vi "GetActivePortNames.vi"(0 "Channel Properties":T1[](array[typedef]) {"Current Pos" format="%.2f"; "Backlash/Eng units" format="%.2f"; "Pulses/rev" format="%.2f"; "Pos Tolerance" format="%.2f"; "Pulses/unit" format="%.2f"; "Acc. Min" format="%.2f"; "Acc. Max" format="%.2f"; "Vel. Min" format="%.2f"; "Vel. Max" format="%.2f"; "Acc. Default" format="%.2f"; "Vel. Default" format="%.2f"}) -> (1 "Port Name Array":string[](array[string]), 2 "Drive Type Array":T2[](array[typedef]), 3 "Address":u8[](array[numeric]))   [LabVIEW 2022 SP3]
uses:
  DriveProperties.ctl
  Traverse Type.ctl
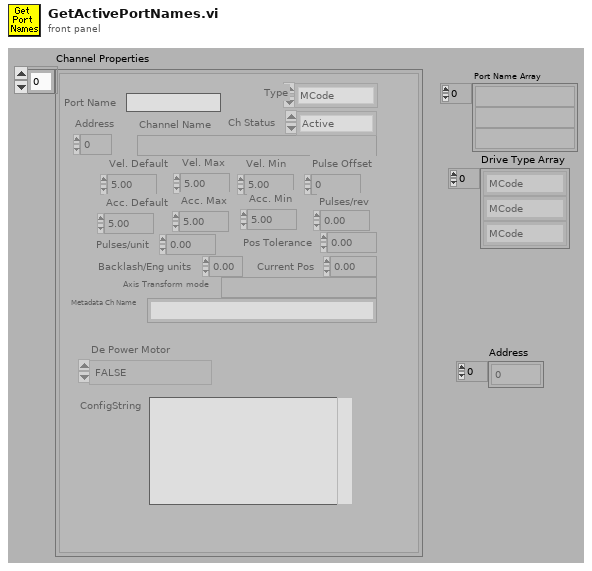
[diagram p1: front panel]
types:
  T1 = typedef "DriveProperties.ctl" = cluster{"Channel Name":string, "Vel. Default":sgl, "Acc. Default":sgl, "Vel. Max":sgl, "Vel. Min":sgl, "Acc. Max":sgl, "Acc. Min":sgl, "Pulses/unit":sgl, "Address":u8, "Pulse Offset":i32, "Pos Tolerance":sgl, "Pulses/rev":sgl, "Backlash/Eng units":sgl, "Current Pos":sgl, "Ch Status":enum16{"Active", "Offline", "Simulate"}, "Port Name":string, "Axis Transform mode":string, "Metadata Ch Name":string, "Type":T2, "De Power Motor":enum16{"TRUE", "FALSE"}, "ConfigString":string}
  T2 = typedef "Traverse Type.ctl" = enum16{"MCode", "Dynamixel"}
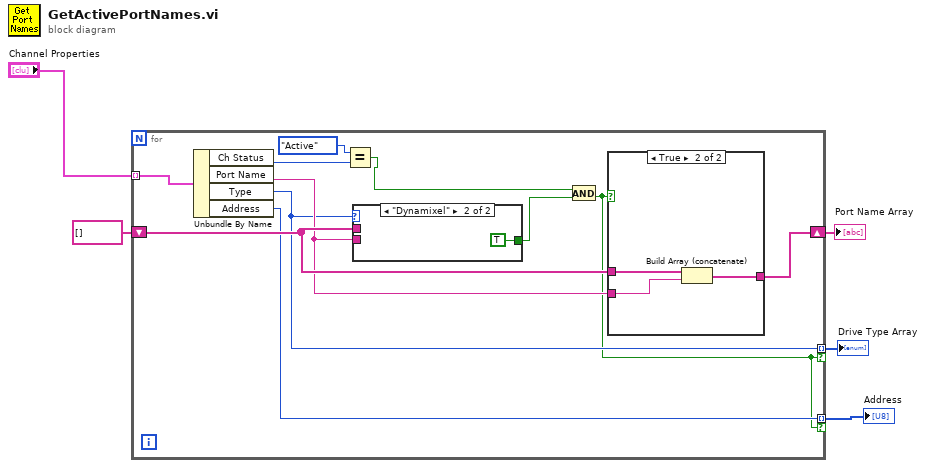
[diagram p0: block diagram]
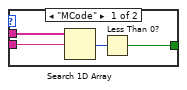
[diagram p2: hidden frame]
diagram:
  n1 = for {
    tunnel: "Channel Properties" -> [w16] mode=indexing
    shift-right: [w13] -> w5
    shift-left: string[] [] -> [w15]
    tunnel: [w8] -> w2 mode=indexing if=w6
    tunnel: [w7] -> w1 mode=indexing if=w6
    n2 = Unbundle By Name(w16) -> ("Ch Status"=w10:enum16{"Active", "Offline", "Simulate"}, "Port Name"=w14:string, "Type"=w8:T2, "Address"=w7:u8)
    n3 = Equal?(x=enum16{"Active", "Offline", "Simulate"}."Active" ("Channel Properties.Ch Status"), y=w10) -> (x = y?=w9:bool)
    n4 = case shown="\"Dynamixel\"" w8 {
      tunnel: w15 -> [w19 _]
      tunnel: w14 -> [w18 _]
      tunnel: [w17 TRUE] -> w12
      frame "MCode" {
        n5 = Search 1D Array(1D array=w19, element=w18) -> (index of element=w20:i32)  [unwired: 1 out]
        n6 = Less Than 0?(x=w20) -> (x < 0?=w17:bool)
      }
      frame "Dynamixel" {
      }
    }
    n7 = And(x=w9, y=w12) -> (x .and. y?=w6:bool)
    n8 = case shown="True" w6 {
      tunnel: w15 -> [w22 w25]
      tunnel: w14 -> [_ w24]
      tunnel: [w22 w23] -> w13
      frame False {
      }
      frame True {
        n9 = Build Array (concatenate)(w25, w24) -> (w23:string[])
      }
    }
  }
  "Port Name Array" <- w5
  "Drive Type Array" <- w2
  "Address" <- w1
